vi "compilingEvent.vi"(8 "error in (no error)":errorcluster, 10 "Path":path, 11 "Compiler in":refnum<class "Compiler.lvclass">) -> (0 "error out":errorcluster, 3 "Compiler out":refnum<class "Compiler.lvclass">)   [LabVIEW 2009, in "Compiler.lvlib" / "Compiler.lvclass"]
uses:
  Compiler.lvclass
  Compiler.lvclass/Compiler.ctl
  Hal/HWController/HWControllerEvents/HWControllerEvents.lvclass
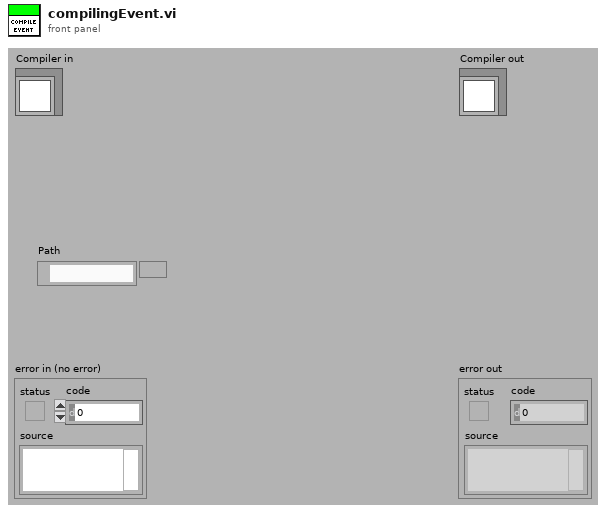
[diagram p1: front panel]
types:
  T1 = enum16{"start", "stop", "statusInquiry", "configure", "resetError", "resourcesInquiry", "reserveResources", "initialise", "resetAllChannels", "staticUpdate", "close", "HWStatus", "error", "resourcesAvailable", "resourcesReserved", "compilerError", "compiledScript", "compilingScript", "runScript", "configureCompiledScript"}
  T2 = cluster{"incomingEventTypes":cluster{"start":cluster{"Boolean":bool}, "stop":cluster{"Boolean":bool}, "statusInquiry":cluster{"Boolean":bool}, "configure":cluster{"DPScriptPath":path, "TimeStamp":string, "HWLoop?":bool}, "resetError":cluster{"Boolean":bool}, "resourcesInquiry":cluster{"Boolean":bool}, "reserveResources":cluster{"HWList":string[]}, "initialise":cluster{"HWList":string[]}, "close":cluster{"Boolean":bool}, "resetAllChannels":cluster{"Boolean":bool}, "staticChannelUpdate":cluster{"channel_address":string, "calibratedValue":dbl}, "runScript":cluster{"DPScriptPath":path, "TimeStamp":string, "HWLoop?":bool}, "compilingScript":cluster{"Path":path}, "compiledScript":cluster{"Path":path, "timeCompileAt":string}, "compilerError":cluster{"Path":path}, "configureCompiledScript":cluster{"DPScriptPath":path, "TimeStamp":string, "HWLoop?":bool, "CompiledScript":cluster{"ScriptListCompiler.lvclass":refnum<class "ScriptListCompiler.lvclass">, "aoChannels":refnum<class "AnalogOutput.lvclass">[], "doChannels":refnum<class "DigitalOutput.lvclass">[], "rfChannels":refnum<class "DDSOutput.lvclass">[]}}, "restartCompiler":cluster{"restart":bool}, "staticRfChannelUpdate":cluster{"channel_address":string, "Output":cluster{"Frequency(MHz)":dbl, "Amplitude":dbl, "Phase":dbl, "OutputForm":enum16{"Sine", "Square", "Triangle", "Arbitrary"}}}, "cameraUpdate":cluster{"Camera":string, "Type":string, "settings":path}}, "outgoingEventTypes":cluster{"HWStatus":cluster{"status":enum16{"Ready", "Compiling", "Configured", "Running", "Stopping", "Unresolved Error"}}, "error":cluster{"error out":errorcluster}, "resourcesAvailable":cluster{"availableHWList":string[], "reservedHWList":string[]}, "resourcesReserved":cluster{"reservedHWList":string[]}}}
  T3 = cluster{"eventId":enum16{"start", "stop", "statusInquiry", "configure", "resetError", "resourcesInquiry", "reserveResources", "initialise", "resetAllChannels", "staticUpdate", "close", "HWStatus", "error", "resourcesAvailable", "resourcesReserved", "compilerError", "compiledScript", "compilingScript", "runScript", "configureCompiledScript"}, "compilingScript":cluster{"Path":path}}
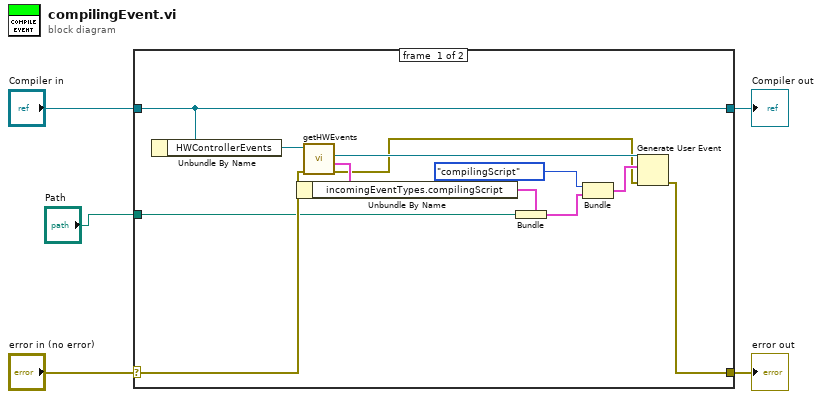
[diagram p0: block diagram]
diagram:
  n1 = case shown="No Error" "error in (no error)" {
    selector: "error in (no error)" -> [w15 w19]
    tunnel: [w6 w19] -> w4
    tunnel: [w17 w18] -> w2
    tunnel: "Compiler in" -> [w17 w18]
    tunnel: "Path" -> [w12 _]
    frame #0 {
      n2 = Unbundle By Name(w17) -> ("HWControllerEvents"=w16:refnum<class "HWControllerEvents.lvclass">)
      n3 = call-dynamic "getHWEvents.vi"("error in (no error)"=w15, "HWControllerEvents in"=w16) -> ("error out"=w7:errorcluster, "eventDataTypes"=w14:T2, "HWCEvent"=w9:refnum<user-event>)  [unwired: 6 in, 1 out]
      n4 = Unbundle By Name(w14) -> ("incomingEventTypes.compilingScript"=w13:cluster{"Path":path})
      n5 = Bundle(cluster=w13, "Path"=w12) -> (w11:cluster{"Path":path})
      n6 = Bundle("eventId"=T1."compilingScript", "compilingScript"=w11) -> (w8:T3)  [unwired: 1 in]
      n7 = Generate User Event(user event=w9, event data cluster=w8, error in=w7) -> (error out=w6:errorcluster)  [unwired: 1 out]
    }
    frame #1 {
    }
  }
  "error out" <- w4
  "Compiler out" <- w2
